vi "AIT 664 Main Page.vi"(8 "error in (no error)":errorcluster, 11 "Node Ptr":T1 format="%.0x") -> (0 "error out":errorcluster)   [LabVIEW 2015, in "AIT 664 Custom Device.lvlib"]
uses:
  AIT 664 Custom Device.lvlib
  <vilib>/NI Veristand/Custom Device API/Custom Device Item Ref.ctl
  Controls and Global/Global.vi
  <vilib>/NI Veristand/Custom Device API/Get Item Property (Path).vi
  <vilib>/NI Veristand/Custom Device API/Get Item Property (String).vi
  <vilib>/NI Veristand/Custom Device API/Set Item Property (String).vi
  <vilib>/NI Veristand/Custom Device API/Custom Device API.lvlib
panel:
  in  "VISA Resource Address":string
  out "Database File":path
  out "MAC Address":string
  out "Network Speed":string
  out "Version":string
  in  "Header":cluster{"Section Name":string}={"Section Name"="AIT 664 Device"}
  in  "Description":string
  out "Name":string
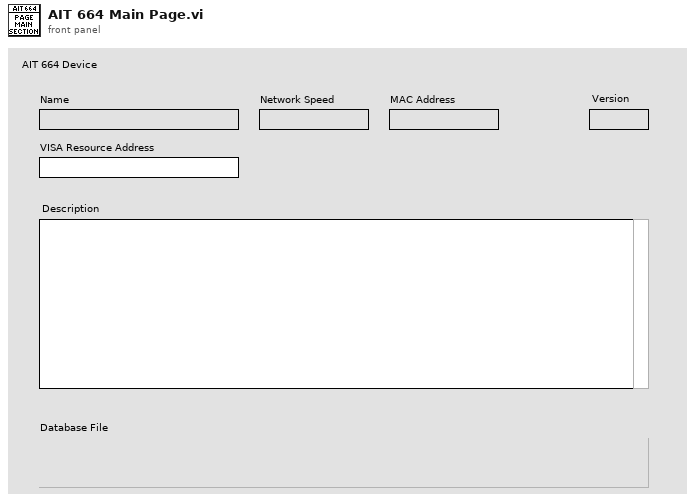
[diagram p1: front panel]
types:
  T1 = typedef "Custom Device API.lvlib/Custom Device Item Ref.ctl" = u64
  T2 = typedef "Custom Device API.lvlib/Custom Device Item Info.ctl" = cluster{"Name":string, "Is Channel":bool, "GUID":string, "Is Waveform":bool}
  T3 = typedef "Custom Device API.lvlib/Custom Device Commands.ctl" = enum16{"Default", "Item renamed", "Shutdown", "Dynamic button pressed"}
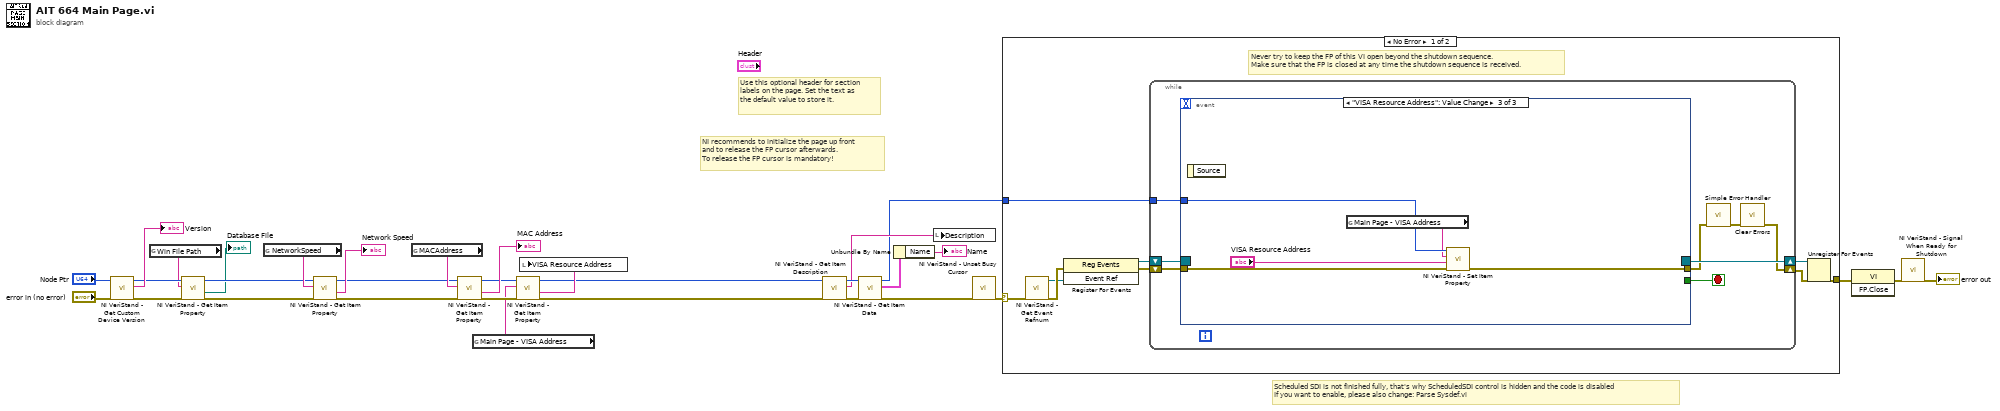
[diagram p0: block diagram]
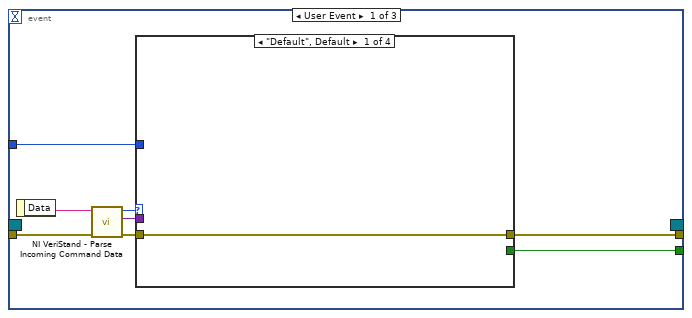
[diagram p2: hidden frame]
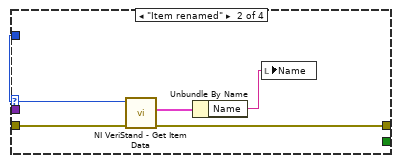
[diagram p3: hidden frame]
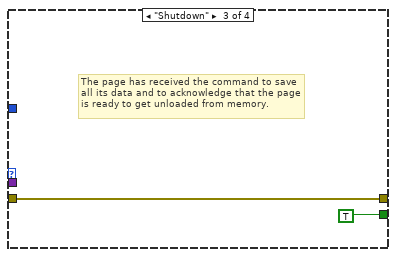
[diagram p4: hidden frame]
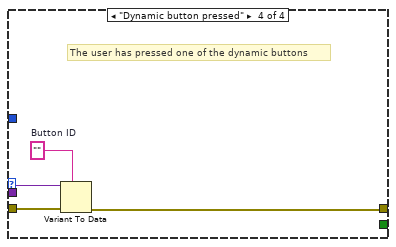
[diagram p5: hidden frame]
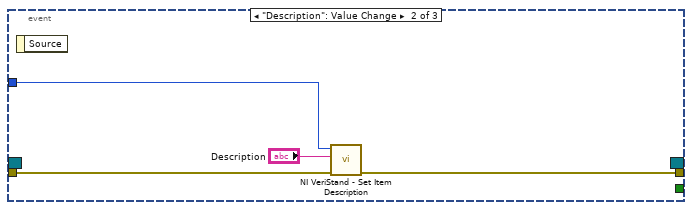
[diagram p6: hidden frame]
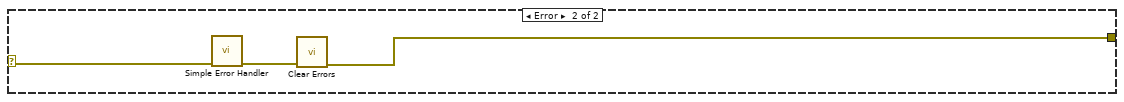
[diagram p7: hidden frame]
diagram:
  # "Scheduled SDI is not finished fully, that's why ScheduledSDI control is hidden and the code is disabled\nIf you want to enable, please also change: Parse Sysdef.vi"
  # "Use this optional header for section labels on the page. Set the text as the default value to store it."
  # "NI recommends to initialize the page up front\nand to release the FP cursor afterwards.\nTo release the FP cursor is mandatory!"
  n1 = call <vilib>:"NI VeriStand - Get Custom Device Version.vi"("error in (no error)"="error in (no error)", "Device Ref in"="Node Ptr") -> ("error out"=w12:errorcluster, "Value"=→"Version":string, "Device Ref out"=w10:T1)  [unwired: 7 in]
  n2 = global read "Global.vi" "Win File Path"() -> (w8:string)
  n3 = call-poly <vilib>:"NI VeriStand - Get Item Property.vi"("error in (no error)"=w12, "Property Name"=w8, "Item Ref in"=w10) -> ("error out"=w11:errorcluster, "Value"=→"Database File":path, "Item Ref out"=w9:T1)  [unwired: 5 in, 1 out]
  n4 = global read "Global.vi" "NetworkSpeed"() -> (w19:string)
  n5 = call-poly <vilib>:"NI VeriStand - Get Item Property.vi"("error in (no error)"=w11, "Property Name"=w19, "Item Ref in"=w9) -> ("error out"=w14:errorcluster, "Value"=→"Network Speed":string, "Item Ref out"=w15:T1)  [unwired: 5 in, 1 out]
  n6 = global read "Global.vi" "MACAddress"() -> (w16:string)
  n7 = call-poly <vilib>:"NI VeriStand - Get Item Property.vi"("error in (no error)"=w14, "Property Name"=w16, "Item Ref in"=w15) -> ("error out"=w5:errorcluster, "Value"=→"MAC Address":string, "Item Ref out"=w6:T1)  [unwired: 5 in, 1 out]
  n8 = global read "Global.vi" "Main Page - VISA Address"() -> (w4:string)
  n9 = call-poly <vilib>:"NI VeriStand - Get Item Property.vi"("error in (no error)"=w5, "Property Name"=w4, "Item Ref in"=w6) -> ("error out"=w1:errorcluster, "Value"=w3:string, "Item Ref out"=w2:T1)  [unwired: 5 in, 1 out]
  n10 = local write "VISA Resource Address"(w3) -> ()
  n11 = call <vilib>:"NI VeriStand - Get Item Description.vi"("error in (no error)"=w1, "Item Ref in"=w2) -> ("error out"=w25:errorcluster, "Description"=w26:string, "Item Ref out"=w27:T1)  [unwired: 7 out]
  n12 = call <vilib>:"NI VeriStand - Get Item Data.vi"("error in (no error)"=w25, "Item Ref in"=w27) -> ("error out"=w29:errorcluster, "Item Info"=w24:T2, "Item Ref out"=w20:T1)  [unwired: 7 out]
  n13 = Unbundle By Name(w24) -> ("Name"=→"Name":string)
  n14 = local write "Description"(w26) -> ()
  n15 = call <vilib>:"NI VeriStand - Unset Busy Cursor.vi"("error in (no error)"=w29) -> ("error out"=w28:errorcluster)  [unwired: 10 out]
  n16 = case shown="No Error" w28 {
    selector: w28 -> [w33 w81]
    tunnel: [w38 w79] -> w32
    tunnel: w20 -> [w34 _]
    frame No Error {
      # "Never try to keep the FP of this VI open beyond the shutdown sequence.\nMake sure that the FP is closed at any time the shutdown sequence is received."
      n17 = call <vilib>:"NI VeriStand - Get Event Refnum.vi"("error in (no error)"=w33) -> ("error out"=w41:errorcluster, "Event Ref"=w37:refnum<user-event>)  [unwired: 9 out]
      n18 = register-events(error in=w41, w37) -> (reference out=w35:refnum<event-registration>, error out=w36:errorcluster)  [unwired: 1 in]
      n19 = while {
        tunnel: w34 -> [w45]
        shift-right: [w42] -> w39
        shift-left: w36 -> [w48]
        shift-right: [w49] -> w40
        shift-left: w35 -> [w47]
        stop <- w46 stop-if-true
        n20 = event shown="[2] \"VISA Resource Address\": Value Change" {
          selector: w47 -> [_ _ _]
          dyn-events: [_ _ _] -> w49
          timeout: _ -> [_ _ _]
          tunnel: w48 -> [w57 w72 w77]
          tunnel: [w53 _ _] -> w46
          tunnel: [w52 w71 w78] -> w44
          tunnel: w45 -> [w51 w73 w76]
          event User Event {
            n21 = event-data() -> ("Data"=w56:string)  [unwired: 1 out]
            n22 = call <vilib>:"NI VeriStand - Parse Incoming Command Data.vi"("error in (no error)"=w57, "Incoming data"=w56) -> ("error out"=w55:errorcluster, "Outgoing data"=w50:variant, "Action"=w54:T3)  [unwired: 7 out]
            n23 = case shown="\"Default\", Default" w54 {
              tunnel: w55 -> [w58 w63 w64 w69]
              tunnel: [_ _ TRUE _] -> w53
              tunnel: [w58 w60 w64 w66] -> w52
              tunnel: w51 -> [_ w62 _ _]
              tunnel: w50 -> [_ _ _ w68]
              frame "Default", Default {
              }
              frame "Item renamed" {
                n24 = call <vilib>:"NI VeriStand - Get Item Data.vi"("error in (no error)"=w63, "Item Ref in"=w62) -> ("error out"=w60:errorcluster, "Item Info"=w61:T2)  [unwired: 8 out]
                n25 = Unbundle By Name(w61) -> ("Name"=w59:string)
                n26 = local write "Name"(w59) -> ()
              }
              frame "Shutdown" {
                # "The page has received the command to save all its data and to acknowledge that the page is ready to get unloaded from memory."
              }
              frame "Dynamic button pressed" {
                w67 = ""  # Button ID
                # "The user has pressed one of the dynamic buttons"
                n27 = Variant To Data(error in=w69, type=w67, Variant=w68) -> (error out=w66:errorcluster)  [unwired: 1 out]
              }
            }
          }
          event "Description": Value Change {
            n28 = event-data() -> ()  [unwired: 2 out]
            n29 = call <vilib>:"NI VeriStand - Set Item Description.vi"("error in (no error)"=w72, "Description"="Description", "Item Ref in"=w73) -> ("error out"=w71:errorcluster)  [unwired: 8 out]
          }
          event "VISA Resource Address": Value Change {
            n30 = event-data() -> ()  [unwired: 2 out]
            n31 = global read "Global.vi" "Main Page - VISA Address"() -> (w74:string)
            n32 = call-poly <vilib>:"NI VeriStand - Set Item Property.vi"("error in (no error)"=w77, "Value"="VISA Resource Address", "Property Name"=w74, "Item Ref in"=w76) -> ("error out"=w78:errorcluster)  [unwired: 5 in, 2 out]
          }
        }
        n33 = call <vilib>:"Simple Error Handler.vi"("error in (no error)"=w44) -> ("error out"=w43:errorcluster)  [unwired: 1 in, 7 out]
        n34 = call <vilib>:"Clear Errors.vi"("error in (no error)"=w43) -> ("error out"=w42:errorcluster)  [unwired: 1 in, 5 out]
      }
      n35 = Unregister For Events(event registration refnum=w40, error in=w39) -> (error out=w38:errorcluster)
    }
    frame Error {
      n36 = call <vilib>:"Simple Error Handler.vi"("error in (no error)"=w81) -> ("error out"=w80:errorcluster)  [unwired: 1 in, 7 out]
      n37 = call <vilib>:"Clear Errors.vi"("error in (no error)"=w80) -> ("error out"=w79:errorcluster)  [unwired: 1 in, 5 out]
    }
  }
  n38 = invoke class="VI" method="FP.Close"(error in=w32) -> (error out=w31:errorcluster)  [unwired: 2 in, 2 out]
  n39 = call <vilib>:"NI VeriStand - Signal When Ready for Shutdown.vi"("error in (no error)"=w31) -> ("error out"=→"error out":errorcluster)  [unwired: 10 out]
